vi "cts_to_cm.vi"(1 "cts":dbl) -> (0 "cm":dbl)   [LabVIEW 2018]
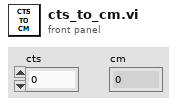
[diagram p1: front panel]
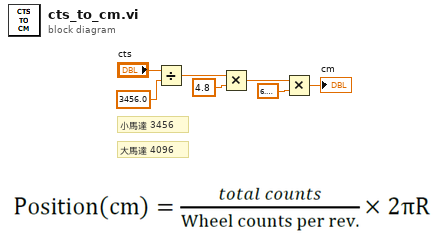
[diagram p0: block diagram]
diagram:
  # "小馬達 3456"
  # "大馬達 4096"
  n1 = Divide(x="cts", y=3456.0) -> (x/y=w5:dbl)
  n2 = Multiply(x=w5, y=4.8 ("x")) -> (x*y=w4:dbl)
  n3 = Multiply(x=w4, y=6.283185307179586) -> (x*y=→"cm":dbl)
